vi "Calculate FPGA Parameters.vi"(5 "Accumulator Size (bit)":i32=32, 6 "Amplitude Scaling Parameters":T1={"Full Scale (V) "=10.0, "Full Scale (binary)"=32768.0}, 7 "Loop Rate (Hz)":dbl, 8 "Signal Offset (V)":dbl=5.0, 9 "Signal Amplitude (V)":dbl=5.0, 10 "Phase Shift (Deg)":dbl, 11 "DDS Signal Frequency (Hz)":dbl=20000.0) -> (0 "AO Offset":i16, 1 "AO Amplitude":u16, 2 "Phase Shift":u32, 3 "Accumulator Increment":u32, 4 "Scaling Ratio":dbl)   [LabVIEW 2017, in "Piezo Controller.lvlib"]
uses:
  Piezo Controller.lvlib
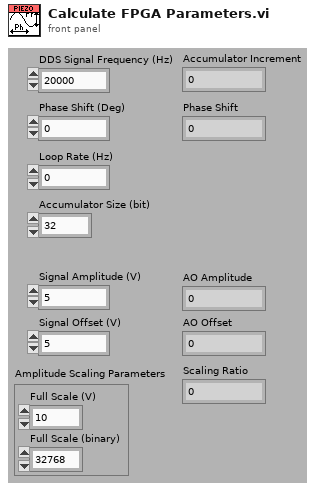
[diagram p1: front panel]
types:
  T1 = cluster{"Full Scale (V) ":dbl, "Full Scale (binary)":dbl}
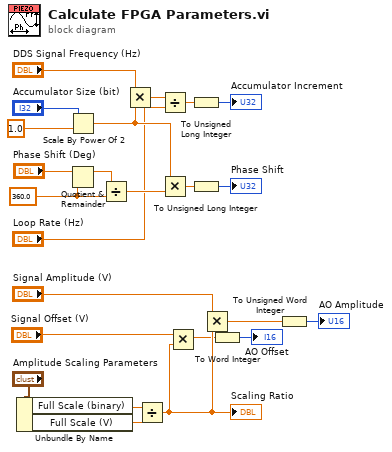
[diagram p0: block diagram]
diagram:
  w6 = 360.0 ("y")
  n1 = Unbundle By Name("Amplitude Scaling Parameters") -> ("Full Scale (binary)"=w11:dbl, "Full Scale (V)"=w10:dbl)
  n2 = Scale By Power Of 2(n="Accumulator Size (bit)", x=1.0) -> (x*2^n=w16:dbl)
  n3 = Quotient & Remainder(x="Phase Shift (Deg)", y=w6) -> (x-y*floor(x/y)=w7:dbl)  [unwired: 1 out]
  n4 = Divide(x=w7, y=w6) -> (x/y=w19:dbl)
  n5 = Multiply(x="DDS Signal Frequency (Hz)", y=w16) -> (x*y=w18:dbl)
  n6 = Divide(x=w11, y=w10) -> (x/y=w4:dbl)
  "Scaling Ratio" <- w4
  n7 = Divide(x=w18, y="Loop Rate (Hz)") -> (x/y=w23:dbl)
  n8 = Multiply(x=w16, y=w19) -> (x*y=w14:dbl)
  n9 = Multiply(x="Signal Offset (V)", y=w4) -> (x*y=w2:dbl)
  n10 = To Unsigned Long Integer(number=w23) -> (unsigned 32bit integer=→"Accumulator Increment":u32)
  n11 = To Unsigned Long Integer(number=w14) -> (unsigned 32bit integer=→"Phase Shift":u32)
  n12 = Multiply(x="Signal Amplitude (V)", y=w4) -> (x*y=w3:dbl)
  n13 = To Word Integer(number=w2) -> (16bit integer=→"AO Offset":i16)
  n14 = To Unsigned Word Integer(number=w3) -> (unsigned 16bit integer=→"AO Amplitude":u16)
